vi "Get Right Position.vi"(11 "drive in":refnum<class "drive.lvclass">) -> (2 "RPosition":dbl, 3 "drive out":refnum<class "drive.lvclass">)   [LabVIEW 2015]
uses:
  drive.lvclass
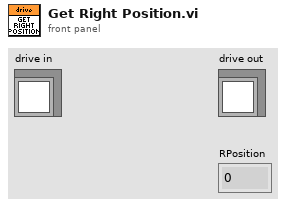
[diagram p1: front panel]
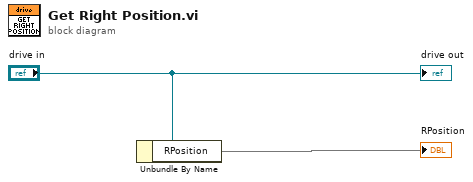
[diagram p0: block diagram]
diagram:
  n1 = Unbundle By Name("drive in") -> ("RPosition"=→"RPosition")
  "drive out" <- "drive in"
